vi "(Sub_VI)_Imp_tabs_AOsignal_generation.vi"(6 "Galvo":T2={"Moving Period(ms)"=3.0, "xArray"=[1.0], "yArray"=[1.0]}, 7 "Laser Pulse":T1={"Pulse Freq"=15.0, "DutyCyle"=32.0, "Volt (power if indicates)"=9.2}, 9 "Stimulation Period (sec)":dbl=1.0, 10 "Base Line Period (sec)":dbl=10.0, 11 "Sampling Freq (KHz)":dbl=20.0) -> (0 "output  array":dbl[][](graph), 1 "yGalvo Signal":dbl[](array[numeric]), 2 "xGalvo Signal":dbl[](array[numeric]), 3 "Laser Pulse":dbl[](array[numeric]))   [LabVIEW 2019]
uses:
  <vilib>/measure/NI_MABase.lvlib
panel:
  in  "Delay (ms)":dbl=1.0
  # "Stimulation Galvo AO signal Generation (for all the IMC tab)\nStimulation Laser AO signal Generation (only for Impulse)"
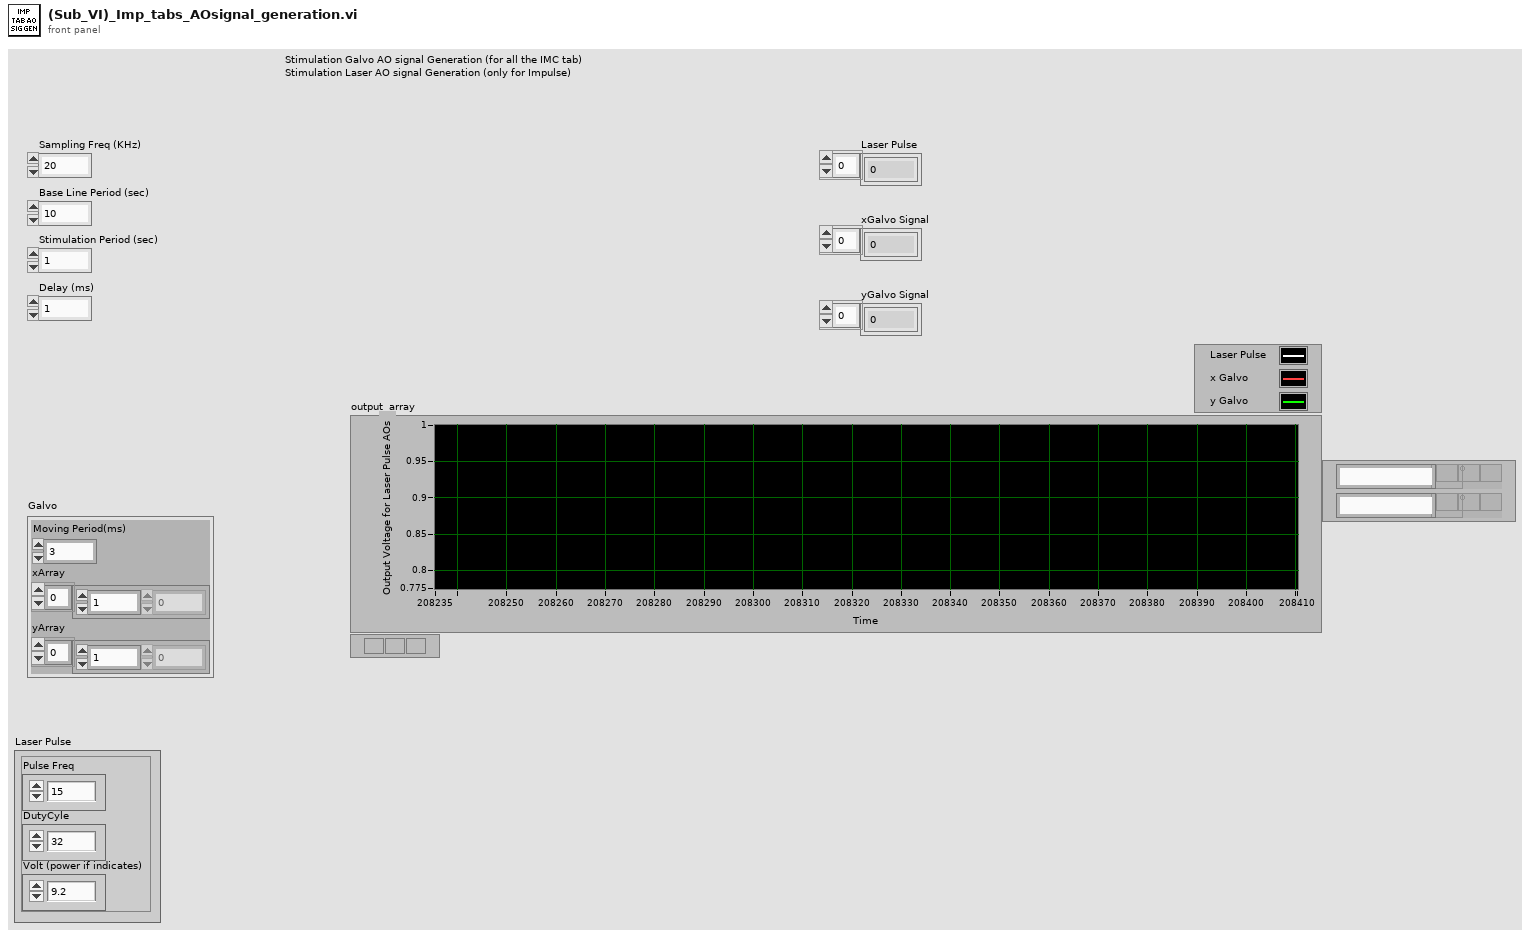
[diagram p1: front panel]
types:
  T1 = cluster{"Pulse Freq":dbl, "DutyCyle":dbl, "Volt (power if indicates)":dbl}
  T2 = cluster{"Moving Period(ms)":dbl, "xArray":dbl[], "yArray":dbl[]}
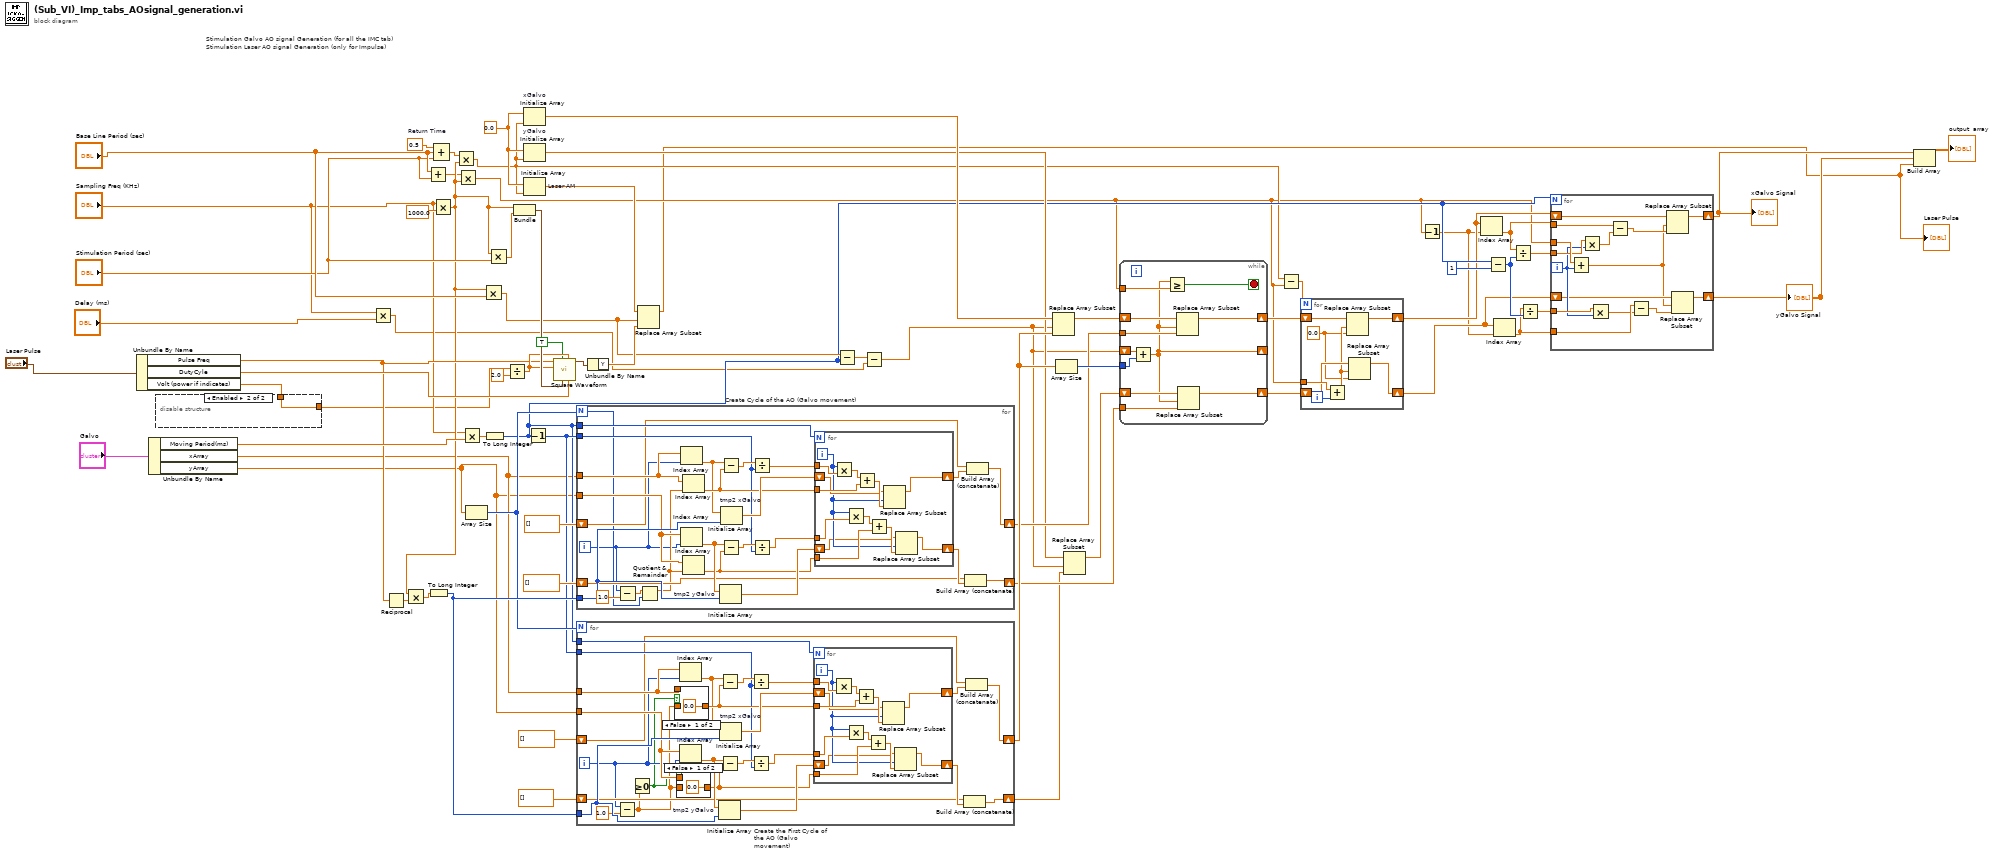
[diagram p0: block diagram]
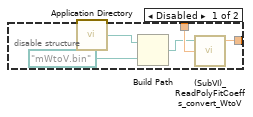
[diagram p2: hidden frame]
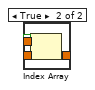
[diagram p3: hidden frame]
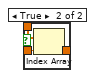
[diagram p4: hidden frame]
diagram:
  w61 = 0.5  # Return Time
  w62 = 0.0 ("element")
  # "Stimulation Galvo AO signal Generation (for all the IMC tab)\nStimulation Laser AO signal Generation (only for Impulse)"
  n1 = Unbundle By Name("Laser Pulse") -> ("Pulse Freq"=w56:dbl, "DutyCyle"=w66:dbl, "Volt (power if indicates)"=w3:dbl)
  n2 = Unbundle By Name("Galvo") -> ("Moving Period(ms)"=w60:dbl, "xArray"=w5:dbl[], "yArray"=w4:dbl[])
  n3 = disable-structure shown="Enabled" {
    disable-tunnel: w3 -> [w73 w75]
    disable-tunnel: [w72 w75] -> w2
    frame Disabled {
      n4 = call <vilib>:"Application Directory.vi"() -> ("Application Directory"=w71:path)
      n5 = Build Path(base path=w71, name or relative path=path "mWtoV.bin" ("file path (use dialog)")) -> (appended path=w70:path)
      n6 = call "(SubVI)_ReadPolyFitCoeffs_convert_WtoV.vi"("Optical Power (mW)"=w73, "file path (use dialog)"=w70) -> ("Voltage (V)"=w72:dbl)  [unwired: 2 in, 1 out]
    }
    frame Enabled {
    }
  }
  n7 = Multiply(x="Sampling Freq (KHz)", y="Delay (ms)") -> (x*y=w8:dbl)
  n8 = Reciprocal(x=w56) -> (1/x=w57:dbl)
  n9 = Add(x="Base Line Period (sec)", y="Stimulation Period (sec)") -> (x+y=w30:dbl)
  n10 = Multiply(x="Sampling Freq (KHz)", y=1000.0) -> (x*y=w31:dbl)
  n11 = Multiply(x=w31, y=w57) -> (x*y=w55:dbl)
  n12 = To Long Integer(number=w55) -> (32bit integer=w51:i32)
  n13 = Compound Arithmetic op=ADD(w61, "Base Line Period (sec)", "Stimulation Period (sec)") -> (w63:dbl)
  n14 = Multiply(x=w63, y=w31) -> (x*y=w20:dbl)
  n15 = Multiply(x=w30, y=w31) -> (x*y=w14:dbl)
  n16 = Multiply(x="Sampling Freq (KHz)", y=w60) -> (x*y=w59:dbl)
  n17 = Array Size(array=w4) -> (size(s)=w50:i32)
  n18 = Multiply(x=w31, y="Base Line Period (sec)") -> (x*y=w44:dbl)
  n19 = To Long Integer(number=w59) -> (32bit integer=w29:i32)
  n20 = Multiply(x=w31, y="Stimulation Period (sec)") -> (x*y=w39:dbl)
  n21 = Divide(x=w2, y=2.0) -> (x/y=w64:dbl)
  n22 = Bundle(w31, w39) -> (w67:cluster{dbl, dbl})  [unwired: 1 in]
  n23 = Initialize Array "xGalvo"(w62, w20) -> (w43:dbl[])
  n24 = Initialize Array "yGalvo"(w62, w20) -> (w37:dbl[])
  n25 = Initialize Array "Laser AM"(w62, w20) -> (w45:dbl[])
  n26 = Decrement(x=w29) -> (x-1=w49:i32)
  n27 = call <vilib>:"Square Waveform.vi"("duty cycle (%)"=w66, "offset"=w64, "sampling info"=w67, "reset signal"=TRUE, "amplitude"=w64, "frequency"=w56) -> ("signal out"=w54:waveform(dbl))  [unwired: 4 in, 1 out]
  n28 = for "Create the First Cycle of the AO (Galvo movement)" {
    N: w50 -> [_]
    tunnel: w29 -> [w100]
    tunnel: w51 -> [w99]
    tunnel: w5 -> [w98]
    tunnel: w4 -> [w91]
    tunnel: w49 -> [w89]
    shift-right: [w83] -> w41
    shift-left: dbl[] [] -> [w85]
    shift-right: [w80] -> w34
    shift-left: dbl[] [] -> [w81]
    i -> [w78]
    n29 = Subtract(x=w78, y=1.0) -> (x-y=w77:dbl)
    n30 = Greater Or Equal To 0?(x=w77) -> (x >= 0?=w76:bool)
    n31 = case shown="False" w76 {
      tunnel: w98 -> [_ w108]
      tunnel: [0.0 w107] -> w94
      tunnel: w77 -> [_ w106]
      frame False {
      }
      frame True {
        n32 = Index Array(array=w108, index=w106) -> (element=w107:dbl)
      }
    }
    n33 = case shown="False" w76 {
      tunnel: w91 -> [_ w104]
      tunnel: [0.0 w103] -> w86
      tunnel: w77 -> [_ w102]
      frame False {
      }
      frame True {
        n34 = Index Array(array=w104, index=w102) -> (element=w103:dbl)
      }
    }
    n35 = Index Array(array=w98, index=w78) -> (element=w93:dbl)
    n36 = Index Array(array=w91, index=w78) -> (element=w88:dbl)
    n37 = Initialize Array "tmp2 yGalvo"(w88, w99) -> (w87:dbl[])
    n38 = Subtract(x=w93, y=w94) -> (x-y=w97:dbl)
    n39 = Initialize Array "tmp2 xGalvo"(w93, w99) -> (w95:dbl[])
    n40 = Subtract(x=w88, y=w86) -> (x-y=w92:dbl)
    n41 = Divide(x=w97, y=w89) -> (x/y=w96:dbl)
    n42 = Divide(x=w92, y=w89) -> (x/y=w90:dbl)
    n43 = for {
      N: w100 -> [_]
      tunnel: w96 -> [w119]
      shift-right: [w116] -> w84
      shift-left: w95 -> [w117]
      tunnel: w94 -> [w121]
      tunnel: w90 -> [w112]
      shift-right: [w113] -> w82
      shift-left: w87 -> [w109]
      tunnel: w86 -> [w111]
      i -> [w110]
      n44 = Multiply(x=w110, y=w119) -> (x*y=w120:dbl)
      n45 = Multiply(x=w110, y=w112) -> (x*y=w115:dbl)
      n46 = Add(x=w120, y=w121) -> (x+y=w118:dbl)
      n47 = Add(x=w115, y=w111) -> (x+y=w114:dbl)
      n48 = Replace Array Subset(array=w117, new element=w118, index=w110) -> (w116:dbl[])
      n49 = Replace Array Subset(array=w109, new element=w114, index=w110) -> (w113:dbl[])
    }
    n50 = Build Array (concatenate)(w81, w82) -> (w80:dbl[])
    n51 = Build Array (concatenate)(w85, w84) -> (w83:dbl[])
  }
  n52 = for "Create Cycle of the AO (Galvo movement)" {
    N: w50 -> [w124]
    tunnel: w29 -> [w147]
    tunnel: w51 -> [w146]
    tunnel: w5 -> [w145]
    tunnel: w4 -> [w138]
    tunnel: w49 -> [w136]
    shift-right: [w130] -> w38
    shift-left: dbl[] [] -> [w132]
    shift-right: [w127] -> w35
    shift-left: dbl[] [] -> [w128]
    i -> [w122]
    n53 = Subtract(x=w122, y=1.0) -> (x-y=w125:dbl)
    n54 = Quotient & Remainder(x=w125, y=w124) -> (x-y*floor(x/y)=w123:dbl)  [unwired: 1 out]
    n55 = Index Array(array=w145, index=w122) -> (element=w140:dbl)
    n56 = Index Array(array=w138, index=w122) -> (element=w135:dbl)
    n57 = Index Array(array=w145, index=w123) -> (element=w141:dbl)
    n58 = Index Array(array=w138, index=w123) -> (element=w133:dbl)
    n59 = Initialize Array "tmp2 yGalvo"(w135, w146) -> (w134:dbl[])
    n60 = Subtract(x=w140, y=w141) -> (x-y=w144:dbl)
    n61 = Initialize Array "tmp2 xGalvo"(w140, w146) -> (w142:dbl[])
    n62 = Subtract(x=w135, y=w133) -> (x-y=w139:dbl)
    n63 = Divide(x=w144, y=w136) -> (x/y=w143:dbl)
    n64 = Divide(x=w139, y=w136) -> (x/y=w137:dbl)
    n65 = for {
      N: w147 -> [_]
      tunnel: w143 -> [w158]
      shift-right: [w155] -> w131
      shift-left: w142 -> [w156]
      tunnel: w141 -> [w160]
      tunnel: w137 -> [w151]
      shift-right: [w152] -> w129
      shift-left: w134 -> [w148]
      tunnel: w133 -> [w150]
      i -> [w149]
      n66 = Multiply(x=w149, y=w158) -> (x*y=w159:dbl)
      n67 = Multiply(x=w149, y=w151) -> (x*y=w154:dbl)
      n68 = Add(x=w159, y=w160) -> (x+y=w157:dbl)
      n69 = Add(x=w154, y=w150) -> (x+y=w153:dbl)
      n70 = Replace Array Subset(array=w156, new element=w157, index=w149) -> (w155:dbl[])
      n71 = Replace Array Subset(array=w148, new element=w153, index=w149) -> (w152:dbl[])
    }
    n72 = Build Array (concatenate)(w128, w129) -> (w127:dbl[])
    n73 = Build Array (concatenate)(w132, w131) -> (w130:dbl[])
  }
  n74 = Unbundle By Name(w54) -> ("Y"=w46:dbl[])
  n75 = Replace Array Subset(array=w45, new element=w46, index=w44) -> (w6:dbl[])
  "Laser Pulse" <- w6
  n76 = Subtract(x=w44, y=w29) -> (x-y=w12:dbl)
  n77 = Subtract(x=w12, y=w8) -> (x-y=w11:dbl)
  n78 = Replace Array Subset(array=w43, new element=w41, index=w11) -> (w42:dbl[])
  n79 = Array Size(array=w41) -> (size(s)=w40:i32)
  n80 = Replace Array Subset(array=w37, new element=w34, index=w11) -> (w36:dbl[])
  n81 = while {
    shift-right: [w165] -> w19
    shift-left: w42 -> [w169]
    tunnel: w40 -> [w167]
    tunnel: w14 -> [w171]
    tunnel: w38 -> [w166]
    shift-right: [w162] -> _
    shift-left: w11 -> [w168]
    shift-right: [w163] -> w17
    shift-left: w36 -> [w164]
    tunnel: w35 -> [w161]
    stop <- w170 stop-if-true
    n82 = Add(x=w168, y=w167) -> (x+y=w162:dbl)
    n83 = Greater Or Equal?(x=w162, y=w171) -> (x >= y?=w170:bool)
    n84 = Replace Array Subset(array=w169, new element=w166, index=w162) -> (w165:dbl[])
    n85 = Replace Array Subset(array=w164, new element=w161, index=w162) -> (w163:dbl[])
  }
  n86 = Subtract(x=w20, y=w14) -> (x-y=w21:dbl)
  n87 = for {
    N: w21 -> [_]
    shift-right: [w176] -> w18
    shift-left: w19 -> [w179]
    shift-right: [w175] -> w16
    shift-left: w17 -> [w174]
    tunnel: w14 -> [w177]
    i -> [w178]
    w172 = 0.0 ("new element/subarray")
    n88 = Add(x=w177, y=w178) -> (x+y=w173:dbl)
    n89 = Replace Array Subset(array=w179, new element=w172, index=w173) -> (w176:dbl[])
    n90 = Replace Array Subset(array=w174, new element=w172, index=w173) -> (w175:dbl[])
  }
  n91 = Decrement(x=w14) -> (x-1=w15:dbl)
  n92 = Index Array(array=w18, index=w15) -> (element=w27:dbl)
  n93 = Subtract(x=w29, y=1) -> (x-y=w26:i32)
  n94 = Index Array(array=w16, index=w15) -> (element=w23:dbl)
  n95 = Divide(x=w27, y=w26) -> (x/y=w25:dbl)
  n96 = Divide(x=w23, y=w26) -> (x/y=w24:dbl)
  n97 = for {
    N: w29 -> [_]
    shift-right: [w184] -> w13
    shift-left: w18 -> [w194]
    tunnel: w14 -> [w193]
    tunnel: w27 -> [w192]
    tunnel: w25 -> [w191]
    tunnel: w24 -> [w188]
    shift-right: [w183] -> w22
    shift-left: w16 -> [w182]
    tunnel: w23 -> [w186]
    i -> [w187]
    n98 = Add(x=w193, y=w187) -> (x+y=w181:dbl)
    n99 = Multiply(x=w191, y=w187) -> (x*y=w190:dbl)
    n100 = Multiply(x=w188, y=w187) -> (x*y=w185:dbl)
    n101 = Subtract(x=w192, y=w190) -> (x-y=w189:dbl)
    n102 = Subtract(x=w186, y=w185) -> (x-y=w180:dbl)
    n103 = Replace Array Subset(array=w194, new element=w189, index=w181) -> (w184:dbl[])
    n104 = Replace Array Subset(array=w182, new element=w180, index=w181) -> (w183:dbl[])
  }
  "xGalvo Signal" <- w13
  "yGalvo Signal" <- w22
  n105 = Build Array(w13, w22, w6) -> (→"output  array":dbl[][])
